vi "Tosca-Save Run.vi"(2 "Notes":refnum<vi>, 7 "Abort?":bool, 9 "Analysis":T2, 11 "error in (no error)":errorcluster, 12 "Session Info":T1={"Animal ID"="", "Session"=1, "Path"=path "", "Run"=0} {"Session" min=1 step=1}) -> (8 "Save data?":bool, 14 "Session Info out":T1={"Animal ID"="", "Session"=1, "Path"=path "", "Run"=0} {"Session" min=1 step=1}, 15 "error out":errorcluster)   [LabVIEW 2020]
uses:
  Typedefs/Tosca-Analysis State.ctl
  Typedefs/Tosca-Adaptation State.ctl
  Typedefs/Tosca-Adaptation Track State.ctl
  Typedefs/Tosca-Adaptation History Element.ctl
  Classes/Parameters/Histogram Data.ctl
  Classes/Parameters/Connect.ctl
  Typedefs/Tosca-Session Info.ctl
  epl-vi-lib/Utility VIs/File IO VIs/Configuration File Wrapper VIs/Config-Write Key (string).vi
  Classes/Parameters/Parameters.lvclass
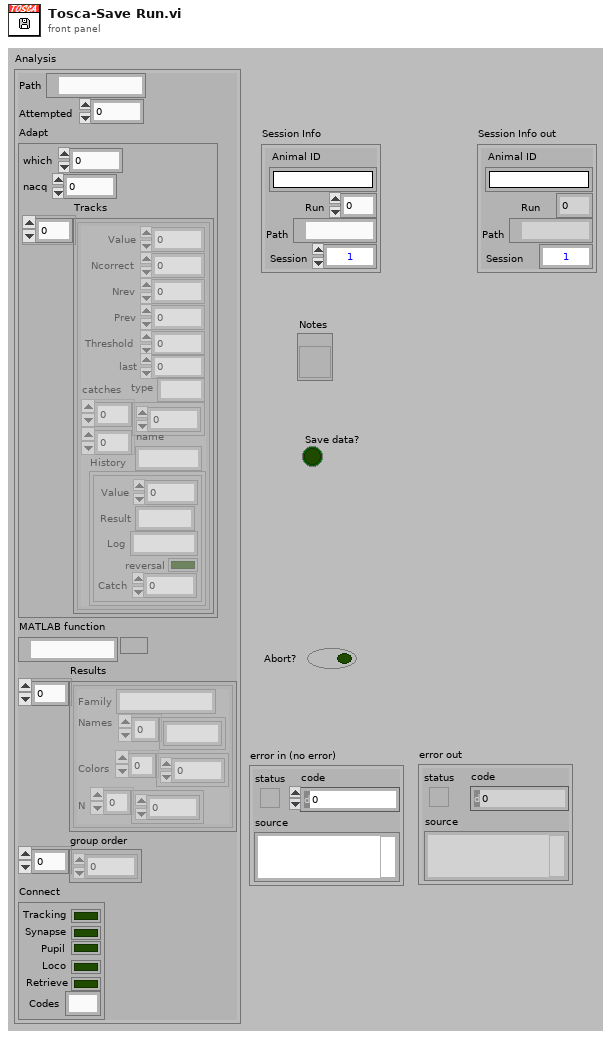
[diagram p1: front panel]
types:
  T1 = typedef "Tosca-Session Info.ctl" = cluster{"Animal ID":string, "Session":i32, "Path":path, "Run":i32}
  T2 = typedef "Tosca-Analysis State.ctl" = cluster{"Path":path, "Attempted":i32, "Adapt":T3, "MATLAB function":path, "Results":T6[], "group order":i32[], "Connect":T7}
  T3 = typedef "Tosca-Adaptation State.ctl" = cluster{"which":i32, "nacq":i32, "Tracks":T4[]}
  T4 = typedef "Tosca-Adaptation Track State.ctl" = cluster{"Value":dbl, "Ncorrect":i32, "Nrev":i32, "Prev":dbl, "History":T5[], "Threshold":dbl, "last":i32, "type":string, "catches":dbl[][], "name":string}
  T5 = typedef "Tosca-Adaptation History Element.ctl" = cluster{"Value":dbl, "Result":string, "Log":string, "reversal":bool, "Catch":dbl}
  T6 = typedef "Parameters.lvclass/Histogram Data.ctl" = cluster{"Family":string, "Names":string[], "Colors":u32[], "N":i32[]}
  T7 = typedef "Parameters.lvclass/Connect.ctl" = cluster{"Tracking":bool, "Synapse":bool, "Pupil":bool, "Loco":bool, "Retrieve":bool, "Codes":string}
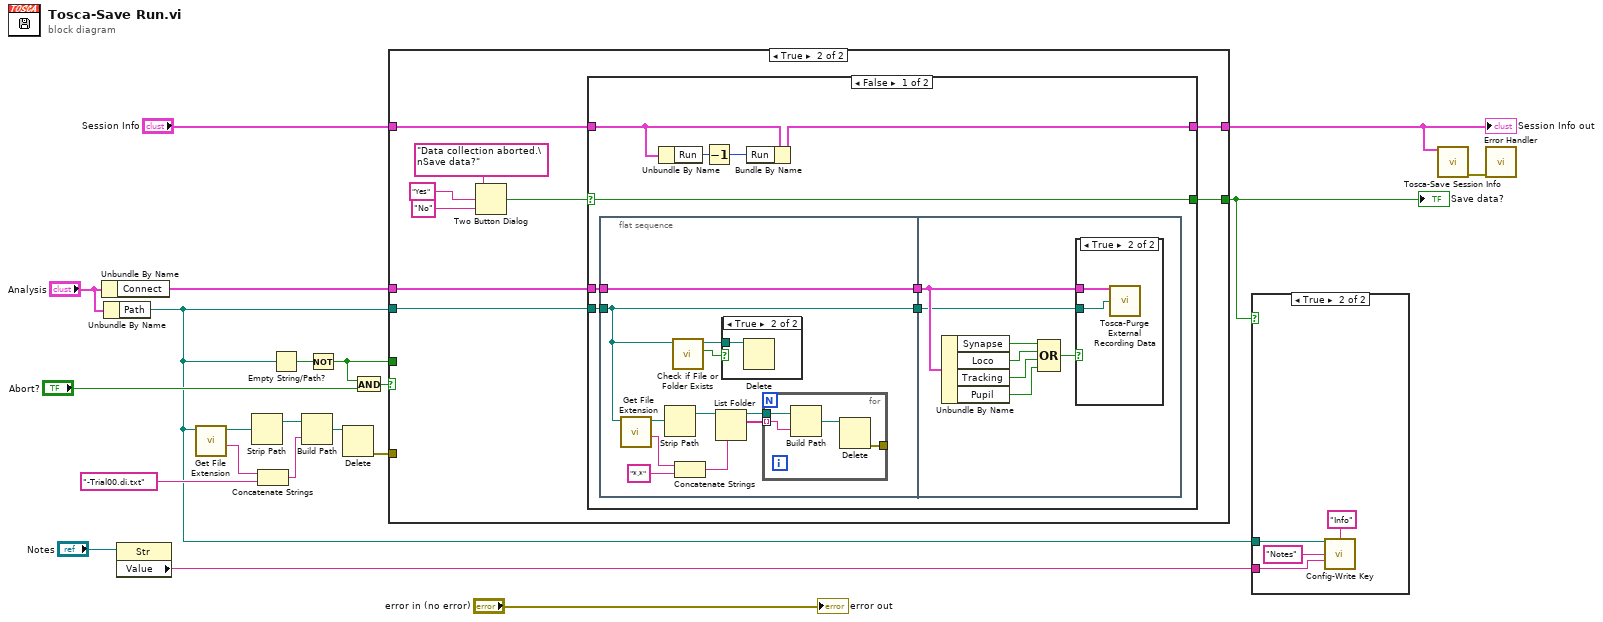
[diagram p0: block diagram]
diagram:
  n1 = Unbundle By Name("Analysis") -> ("Connect"=w1:T7)
  n2 = Unbundle By Name("Analysis") -> ("Path"=w5:path)
  n3 = property class="Str"(reference="Notes") -> ("Value"=w3:string)  [unwired: 1 in, 2 out]
  n4 = call <vilib>:"Get File Extension.vi"("file"=w5) -> ("filename without extension"=w12:string, "dup file"=w8:path)  [unwired: 6 in, 3 out]
  n5 = Strip Path(path=w8) -> (stripped path=w7:path)  [unwired: 1 out]
  n6 = Concatenate Strings(w12, "-Trial00.di.txt" ("string")) -> (w10:string)
  n7 = Empty String/Path?(string/path=w5) -> (empty?=w16:bool)
  n8 = Build Path(base path=w7, name or relative path=w10) -> (appended path=w9:path)
  n9 = Not(x=w16) -> (.not. x?=w15:bool)
  n10 = Delete(path (use dialog)=w9) -> (error out=w13:errorcluster)  [unwired: 4 in, 2 out]
  n11 = And(x=w15, y="Abort?") -> (x .and. y?=w17:bool)
  n12 = case shown="True" w17 {
    tunnel: "Session Info" -> [w23 w28]
    tunnel: [w23 w27] -> w19
    tunnel: [w22 w26] -> w6
    tunnel: w5 -> [_ w25]
    tunnel: w15 -> [w22 _]
    tunnel: w13 -> [_ _]
    tunnel: w1 -> [_ w24]
    frame False {
    }
    frame True {
      n13 = Two Button Dialog(message="Data collection aborted.\nSave data?", 1:"No" ("F button name (\"Cancel\")"), 2:"Yes" ("T button name (\"OK\")")) -> (T button?=w29:bool)
      n14 = case shown="False" w29 {
        selector: w29 -> [w37 w67]
        tunnel: w25 -> [w36 _]
        tunnel: w28 -> [w39 w68]
        tunnel: [w38 w68] -> w27
        tunnel: [w37 w67] -> w26
        tunnel: w24 -> [w34 _]
        frame False {
          n15 = flat-sequence {
            tunnel: w36 -> [w42]
            tunnel: [w43] -> w35
            tunnel: w34 -> [w43]
            tunnel: [w42] -> w33
            tunnel: w35 -> [w59]
            tunnel: w33 -> [w58]
            frame #0 {
              n16 = call <vilib>:"Get File Extension.vi"("file"=w42) -> ("filename without extension"=w49:string, "dup file"=w50:path)  [unwired: 6 in, 3 out]
              n17 = Strip Path(path=w50) -> (stripped path=w47:path)  [unwired: 1 out]
              n18 = call <vilib>:"Check if File or Folder Exists.vi"("path"=w42) -> ("file or folder exists?"=w51:bool, "dup path"=w52:path)  [unwired: 8 in, 1 out]
              n19 = Concatenate Strings(w49, "*.*" ("string")) -> (w46:string)
              n20 = List Folder(path=w47, pattern=w46) -> (path out=w44:path, filenames=w45:string[])  [unwired: 2 in, 2 out]
              n21 = case shown="True" w51 {
                tunnel: w52 -> [_ w57]
                frame False {
                }
                frame True {
                  n22 = Delete(path (use dialog)=w57) -> ()  [unwired: 4 in, 3 out]
                }
              }
              n23 = for {
                tunnel: w45 -> [w55] mode=indexing
                tunnel: w44 -> [w56]
                tunnel: [w53] -> _
                n24 = Build Path(base path=w56, name or relative path=w55) -> (appended path=w54:path)
                n25 = Delete(path (use dialog)=w54) -> (error out=w53:errorcluster)  [unwired: 4 in, 2 out]
              }
            }
            frame #1 {
              n26 = Unbundle By Name(w59) -> ("Synapse"=w64:bool, "Loco"=w63:bool, "Tracking"=w62:bool, "Pupil"=w61:bool)
              n27 = Compound Arithmetic op=OR(w64, w63, w62, w61) -> (w60:bool)
              n28 = case shown="True" w60 {
                tunnel: w59 -> [_ w66]
                tunnel: w58 -> [_ w65]
                frame False {
                }
                frame True {
                  n29 = call "Tosca-Purge External Recording Data.vi"("Connect"=w66, "Path"=w65) -> ()  [unwired: 13 in, 1 out]
                }
              }
            }
          }
          n30 = Unbundle By Name(w39) -> ("Run"=w41:i32)
          n31 = Decrement(x=w41) -> (x-1=w40:i32)
          n32 = Bundle By Name(cluster=w39, "Run"=w40) -> (w38:T1)
        }
        frame True {
        }
      }
    }
  }
  "Session Info out" <- w19
  "Save data?" <- w6
  n33 = case shown="True" w6 {
    tunnel: w5 -> [_ w72]
    tunnel: w3 -> [_ w69]
    frame False {
    }
    frame True {
      n34 = call-poly "Config-Write Key.vi"("configuration file path"=w72, "section"="Info", "key"="Notes", "value"=w69) -> ()  [unwired: 9 in, 3 out]
    }
  }
  n35 = call "Tosca-Save Session Info.vi"("Session Info"=w19) -> ("error out"=w18:errorcluster)  [unwired: 14 in]
  n36 = call "Error Handler.vi"("error in (no error)"=w18) -> ()  [unwired: 12 in, 3 out]
  "error out" <- "error in (no error)"
